vi "Initialise.vi"(8 "error in (no error)":errorcluster, 10 "Actors":refnum<vi>, 11 "Actor in":refnum<class "Debugger.lvclass">) -> (0 "error out":errorcluster, 3 "Actor out":refnum<class "Debugger.lvclass">, 5 "Observers":cluster{"Actor":refnum<event-registration>})   [LabVIEW 2015, in "Debugger.lvclass"]
uses:
  Debugger.lvclass
  Messaging/Message/Message.lvclass
  Debugger.lvclass/Debugger.ctl
  Utility/Utility.lvlib
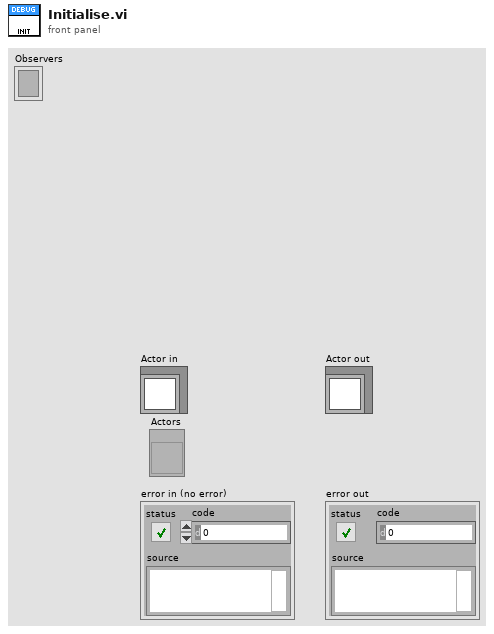
[diagram p1: front panel]
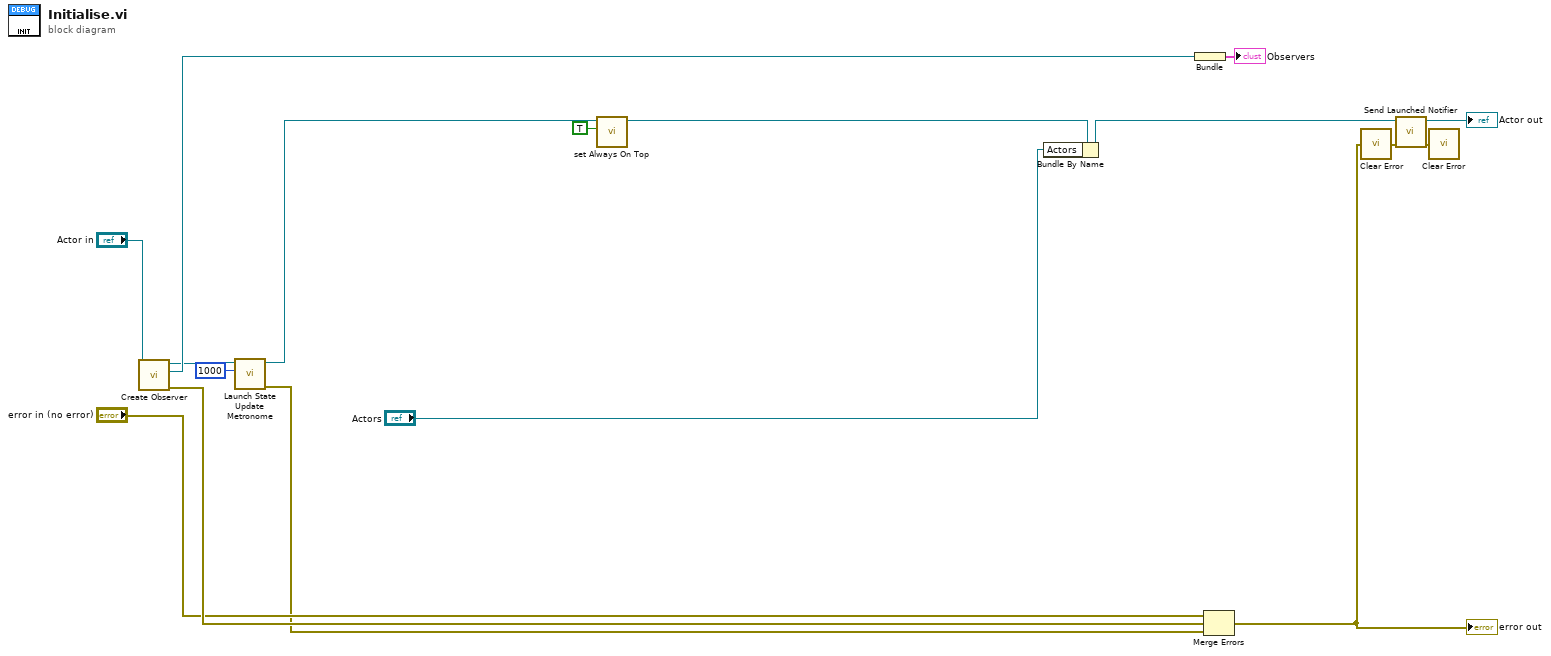
[diagram p0: block diagram]
diagram:
  n1 = call-dynamic "Create Observer.vi"("Actor in"="Actor in") -> ("error out"=w15:errorcluster, "Actor"=w10:refnum<event-registration>, "Actor out"=w8:refnum<class "Debugger.lvclass">)  [unwired: 8 in]
  n2 = call-dynamic "Launch State Update Metronome.vi"("Status Update Period [1000 ms]"=1000, "Actor in"=w8) -> ("error out"=w6:errorcluster, "Actor out"=w3:refnum<class "Debugger.lvclass">)  [unwired: 8 in]
  n3 = call-dynamic "set Always On Top.vi"("Always On Top"=TRUE, "Actor in"=w3) -> ("Actor out"=w2:refnum<class "Debugger.lvclass">)  [unwired: 8 in, 1 out]
  n4 = Bundle By Name(cluster=w2, "Actors"="Actors") -> (w5:refnum<class "Debugger.lvclass">)
  n5 = Bundle("Actor"=w10) -> (→"Observers":cluster{"Actor":refnum<event-registration>})  [unwired: 1 in]
  n6 = Merge Errors("error in (no error)", w15, w6) -> (w14:errorcluster)
  "error out" <- w14
  n7 = call "Clear Error.vi"("error in (no error)"=w14) -> ("error out"=w13:errorcluster)
  n8 = call-dynamic "Send Launched Notifier.vi"("error in (no error)"=w13, "Actor in"=w5) -> ("error out"=w12:errorcluster, "Actor out"=→"Actor out":refnum<class "Debugger.lvclass">)  [unwired: 8 in]
  n9 = call "Clear Error.vi"("error in (no error)"=w12) -> ()  [unwired: 1 out]
